vi "SL2_AD_DLL_Phoibos_GetVoltage.vi"(6 "error in":errorcluster, 7 "voltage_name":string, 8 "pHandle":u32, 9 "dll path in":path) -> (0 "error out":errorcluster, 1 "value":dbl, 3 "dll path out":path)   [LabVIEW 2020]
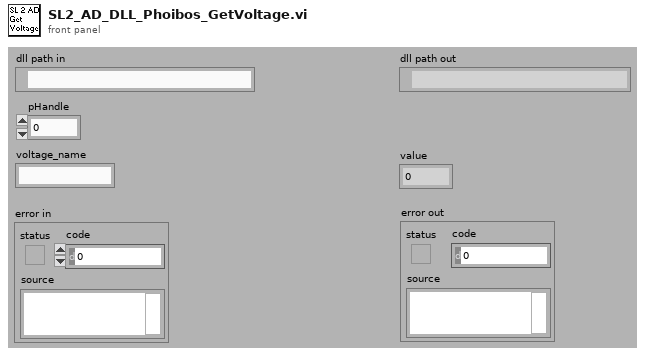
[diagram p1: front panel]
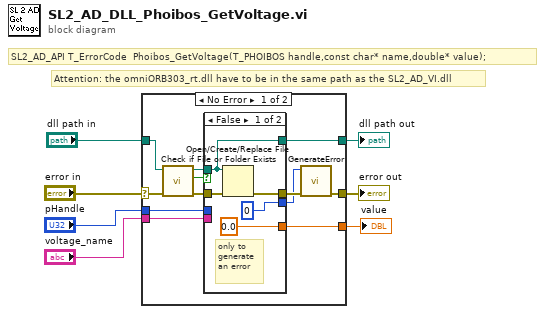
[diagram p0: block diagram]
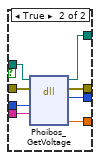
[diagram p2: hidden frame]
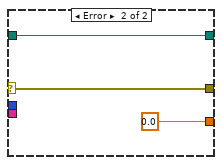
[diagram p3: hidden frame]
diagram:
  # "SL2_AD_API T_ErrorCode  Phoibos_GetVoltage(T_PHOIBOS handle,const char* name,double* value);"
  # "Attention: the omniORB303_rt.dll have to be in the same path as the SL2_AD_VI.dll"
  n1 = case shown="No Error" "error in" {
    selector: "error in" -> [w18 w34]
    tunnel: [w12 w34] -> w7
    tunnel: [w19 w35] -> w6
    tunnel: "dll path in" -> [w17 w35]
    tunnel: "voltage_name" -> [w16 _]
    tunnel: "pHandle" -> [w15 _]
    tunnel: [w14 0.0 ("max")] -> w1
    frame No Error {
      n2 = call <vilib>:"Check if File or Folder Exists.vi"("error in (no error)"=w18, "path"=w17) -> ("error out"=w8:errorcluster, "file or folder exists?"=w10:bool, "dup path"=w9:path)  [unwired: 7 in]
      n3 = case shown="False" w10 {
        tunnel: [w23 w32] -> w13
        tunnel: [u32 0 ("error_code") w31] -> w11
        tunnel: [w22 w30] -> w19
        tunnel: w9 -> [w22 w29]
        tunnel: w8 -> [w24 w28]
        tunnel: w16 -> [_ w27]
        tunnel: w15 -> [_ w26]
        tunnel: [0.0 ("min") w25] -> w14
        frame False {
          # "only to generate an error"
          n4 = Open/Create/Replace File(file path (use dialog)=w22, error in=w24) -> (error out=w23:errorcluster)  [unwired: 4 in, 2 out]
        }
        frame True {
          n5 = dll-call lib="C:/Programme/SPECS/SpecsLab2/programming/LabView7.1/SL2_AD_VI.dll" fn="Phoibos_GetVoltage" ("GetVoltageRange")(path in=w29, error in=w28, "handle"=w26, "voltage_name"=w27) -> (path out=w30:path, error out=w32:errorcluster, "error_code"=w31:u32, "value"=w25:dbl)  [unwired: 4 in]
        }
      }
      n6 = call "GenerateError.vi"("error in"=w13, "error_code"=w11) -> ("error out"=w12:errorcluster)  [unwired: 9 in]
    }
    frame Error {
    }
  }
  "error out" <- w7
  "dll path out" <- w6
  "value" <- w1
